vi "labview.vi"() -> ()   [LabVIEW 2020]
uses:
  <vilib>/Instr/_visa.llb/VISA Configure Serial Port (Instr).vi
panel:
  out "Alarm":bool
  out "Status":dbl
  out "Preesure":dbl(graph)
  out "Humidity":dbl(graph)
  out "Temperature":dbl(graph)
  out "Data":dbl[](array[numeric])
  in  "Stop":bool
  in  "VISA resource name":refnum<visa-resource-name>
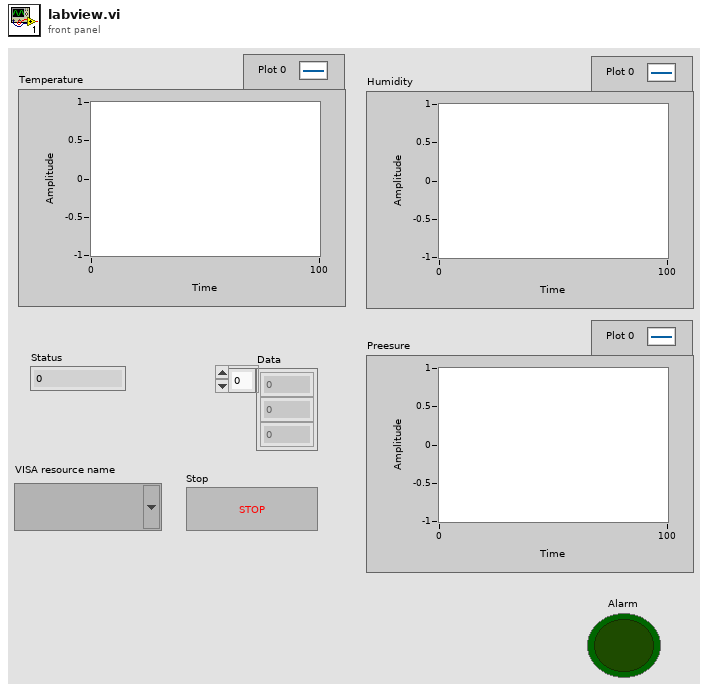
[diagram p1: front panel]
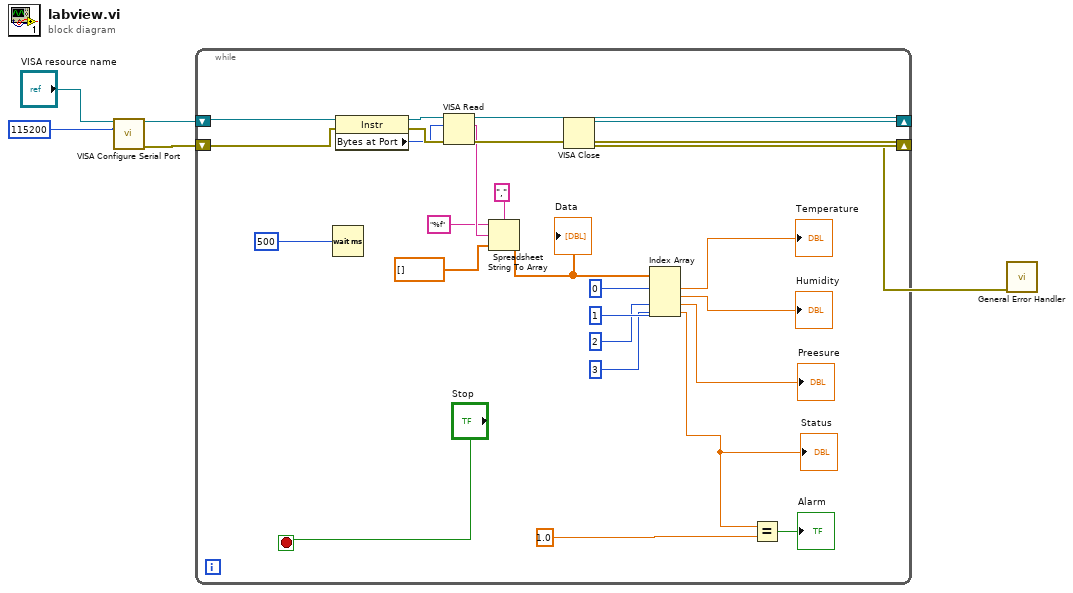
[diagram p0: block diagram]
diagram:
  n1 = call-poly "VISA Configure Serial Port"("VISA resource name"="VISA resource name", "baud rate (9600)"=u32 115200) -> ("VISA resource name out"=w5:refnum<visa-resource-name>, "error out"=w4:errorcluster)  [unwired: 12 in]
  n2 = while {
    shift-right: [w25] -> w3
    shift-left: w5 -> [w13]
    shift-right: [w28] -> w2
    shift-left: w4 -> [w12]
    stop <- "Stop" stop-if-true
    n3 = Wait (ms)(milliseconds to wait=u32 500) -> ()  [unwired: 1 out]
    n4 = property class="Instr"(reference=w13, error in=w12) -> (reference out=w31:refnum<visa-resource-name>, error out=w30:errorcluster, "Bytes at Port"=w29:u32)
    n5 = VISA Read(VISA resource name=w31, byte count=w29, error in (no error)=w30) -> (VISA resource name out=w25:refnum<visa-resource-name>, read buffer=w23:string, error out=w28:errorcluster)  [unwired: 1 out]
    n6 = Spreadsheet String To Array(delimiter (Tab)=",", format string="%f", spreadsheet string=w23, array type (2D Dbl)=dbl[] []) -> (array=w20:dbl[])
    "Data" <- w20
    n7 = Index Array(array=w20, index #1=0 ("index"), index #2=1 ("index"), index #3=2 ("index"), index #4=3 ("index")) -> (element #1=→"Temperature":dbl, element #2=→"Humidity":dbl, element #3=→"Preesure":dbl, element #4=w10:dbl)
    "Status" <- w10
    n8 = Equal?(x=w10, y=1.0) -> (x = y?=→"Alarm":bool)
  }
  n9 = VISA Close(VISA resource name=w3, error in (no error)=w2) -> (error out=w1:errorcluster)
  n10 = call <vilib>:"General Error Handler.vi"("error in (no error)"=w1) -> ()  [unwired: 10 in, 5 out]
